vi "Power Keep Sign (simpler).vi"(1 "Power":dbl, 2 "In":dbl) -> (0 "Out":dbl)   [LabVIEW 2013]
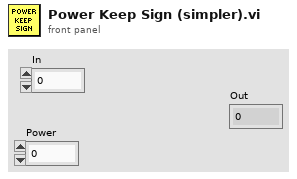
[diagram p1: front panel]
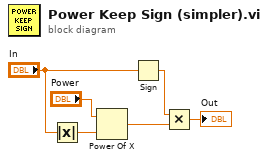
[diagram p0: block diagram]
diagram:
  n1 = Absolute Value(x="In") -> (abs(x)=w5:dbl)
  n2 = Power Of X(1:w5, 2:"Power") -> (0:w1:dbl)
  n3 = Sign(1:"In") -> (0:w3:dbl)
  n4 = Multiply(x=w3, y=w1) -> (x*y=→"Out":dbl)
